vi "Boolean to JSON element.vi"(10 "boolean":bool, 11 "keyword":string) -> (2 "JSON last element":string, 3 "JSON element":string)   [LabVIEW 2012]
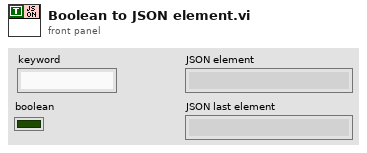
[diagram p1: front panel]
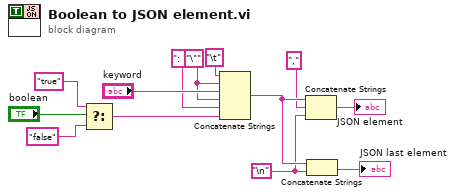
[diagram p0: block diagram]
diagram:
  w2 = "\n"
  w11 = "\""
  n1 = Select(t="true", s="boolean", f="false") -> (s? t:f=w7:string)
  n2 = Concatenate Strings("\t", w11, "keyword", w11, ": ", w7) -> (w4:string)
  n3 = Concatenate Strings(w4, ",", w2) -> (→"JSON element":string)
  n4 = Concatenate Strings(w4, w2) -> (→"JSON last element":string)
